vi "setName.vi"(0 "reference":refnum<class "FinalStateNode.lvclass">, 1 "name":refnum<class "MultiLineString.lvclass">, 5 "error in (no error)":errorcluster) -> (14 "reference out":refnum<class "FinalStateNode.lvclass">, 19 "error out":errorcluster)   [LabVIEW 2016, in "FinalStateNode.lvclass"]
doc: "public void setName(MultiLineString newValue)"
uses:
  <resource>/Framework/Providers/Open_GDS/UML/FinalStateNode_class/FinalStateNode.lvclass
  <resource>/Framework/Providers/Open_GDS/UML/MultiLineString_class/MultiLineString.lvclass
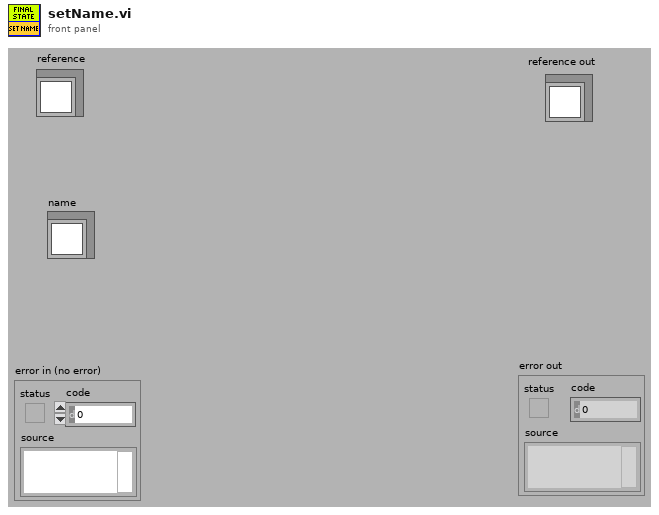
[diagram p1: front panel]
types:
  T1 = typedef "FinalStateNode.lvclass/ObjectAttributes.ctl" = cluster{"name":refnum<class "MultiLineString.lvclass">, "DEFAULT_WIDTH":i32, "DEFAULT_HEIGHT":i32}
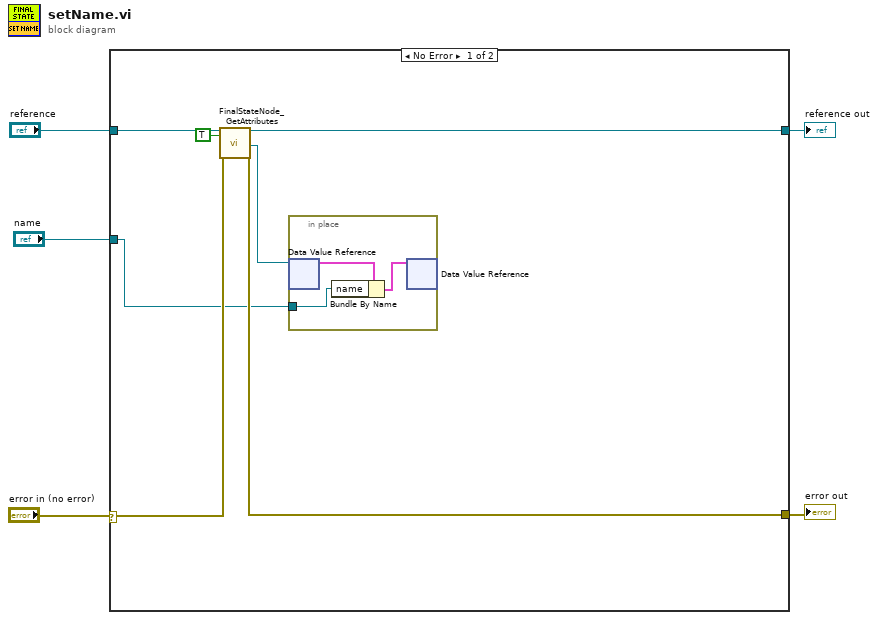
[diagram p0: block diagram]
diagram:
  n1 = case shown="No Error" "error in (no error)" {
    selector: "error in (no error)" -> [w10 w16]
    tunnel: "reference" -> [w12 w17]
    tunnel: [w11 w16] -> w4
    tunnel: [w6 w17] -> w3
    tunnel: "name" -> [w7 _]
    frame No Error {
      n2 = call <resource>:"FinalStateNode_GetAttributes.vi"("reference in"=w12, "OnlyGetDvrReference(False)"=TRUE, "error in (no error)"=w10) -> ("reference out"=w6:refnum<class "FinalStateNode.lvclass">, "DataRef"=w8:refnum<data-value>, "error out"=w11:errorcluster)  [unwired: 13 in, 1 out]
      n3 = in-place {
        in-place-border: w7 -> [w14]
        n4 = in-place-dvr #1(w8) -> (w15:T1)  [unwired: 1 out]
        n5 = Bundle By Name(cluster=w15, "name"=w14) -> (w13:T1)
        n6 = in-place-dvr #1(w13) -> ()  [unwired: 2 out]
      }
    }
    frame Error {
    }
  }
  "reference out" <- w3
  "error out" <- w4
